vi "JogCw.vi"(8 "error in (no error)":errorcluster, 11 "Motor in":refnum<class "Motor.lvclass">) -> (0 "error out":errorcluster, 2 "Response from Controlador":string, 3 "Motor out":refnum<class "Motor.lvclass">)   [LabVIEW 2012, in "Motor.lvclass"]
uses:
  Motor.lvclass
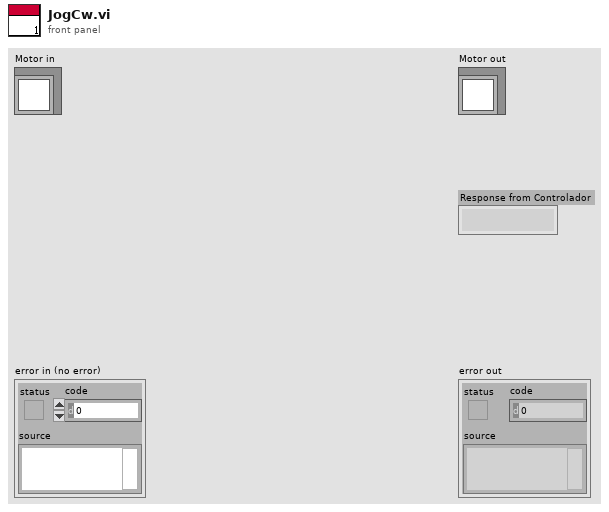
[diagram p1: front panel]
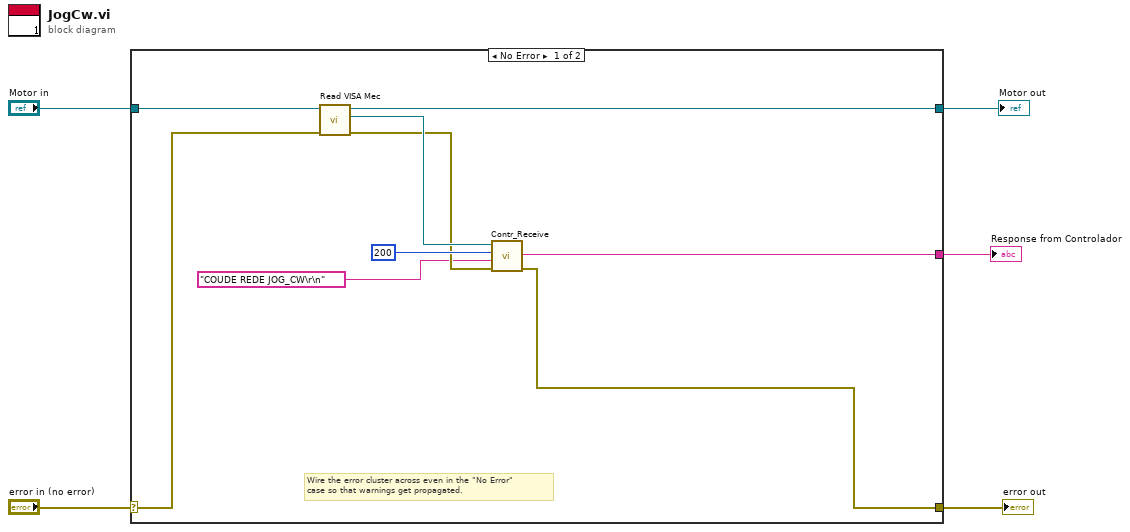
[diagram p0: block diagram]
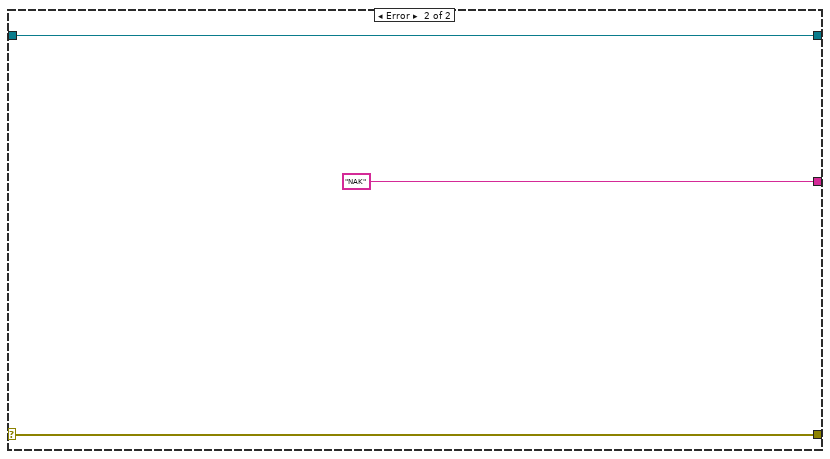
[diagram p2: hidden frame]
diagram:
  n1 = case shown="No Error" "error in (no error)" {
    selector: "error in (no error)" -> [w10 w17]
    tunnel: [w7 w17] -> w4
    tunnel: [w11 w16] -> w2
    tunnel: "Motor in" -> [w12 w16]
    tunnel: [w6 "NAK" ("Response from SIFS")] -> w1
    frame No Error {
      # "Wire the error cluster across even in the \"No Error\"\ncase so that warnings get propagated."
      n2 = call-dynamic "Read VISA Mec.vi"("error in (no error)"=w10, "Controlador in"=w12) -> ("error out"=w9:errorcluster, "VISA Mec"=w13:refnum<visa-resource-name>, "Controlador out"=w11:refnum<class "Motor.lvclass">)  [unwired: 7 in]
      n3 = call "Contr_Receive.vi"("error in"=w9, "Command to SIFS"="COUDE REDE JOG_CW\r\n", "wait after tx"=u32 200, "VISA resource name"=w13) -> ("error out"=w7:errorcluster, "Response from SIFS"=w6:string)  [unwired: 2 out]
    }
    frame Error {
    }
  }
  "error out" <- w4
  "Motor out" <- w2
  "Response from Controlador" <- w1
